vi "SSL UDP Receiver.vi"(11 "Cluster":T1) -> (0 "error out":errorcluster, 2 "RX":bool, 3 "data camera out":u8[](array[numeric]))   [LabVIEW 2020]
uses:
  Controls/vision_control.ctl
  <vilib>/Utility/tcp.llb/UDP Multicast Read-Only Open.vi
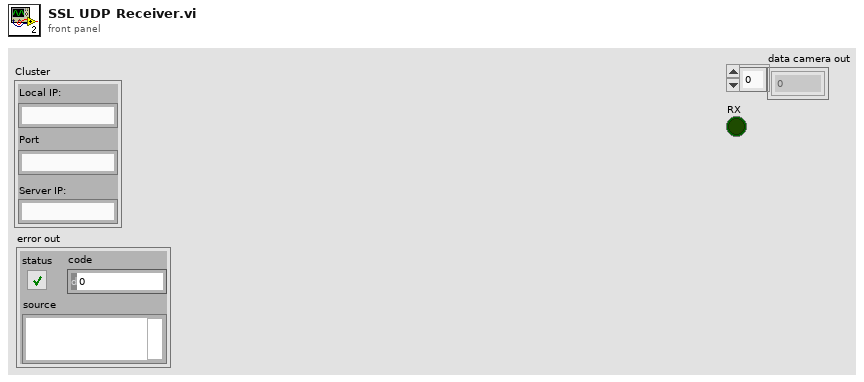
[diagram p1: front panel]
types:
  T1 = typedef "vision_control.ctl" = cluster{"Local IP:":string, "Server IP:":string, "Port":string}
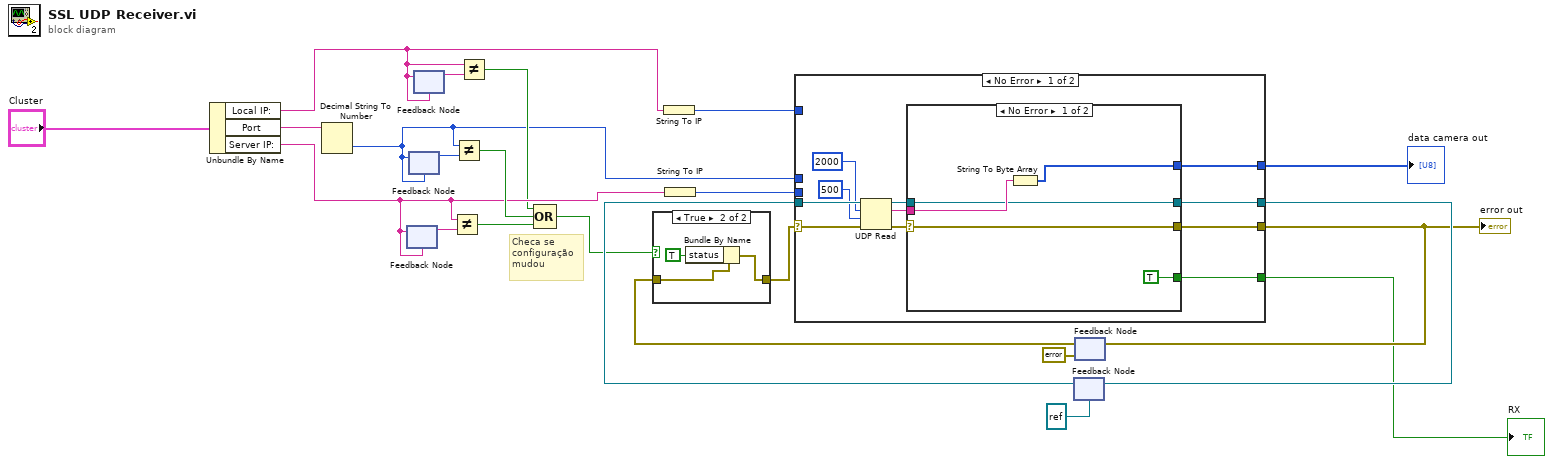
[diagram p0: block diagram]
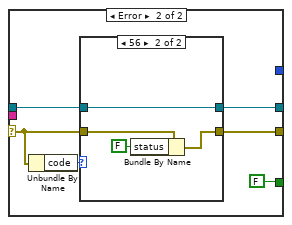
[diagram p3: hidden frame]
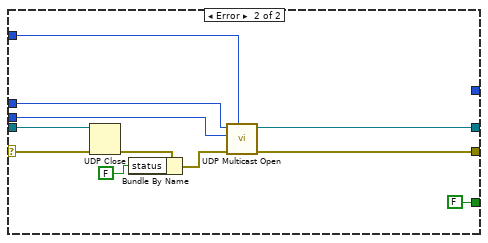
[diagram p5: hidden frame]
diagram:
  # "Checa se \nconfiguração\nmudou"
  n1 = Unbundle By Name("Cluster") -> ("Local IP:"=w8:string, "Port"=w2:string, "Server IP:"=w11:string)
  n2 = Decimal String To Number(string=w2) -> (number=w1:i32)  [unwired: 2 in, 1 out]
  n3 = feedback-in #1(w11) -> ()
  n4 = feedback #1(w11) -> (w16:string)
  n5 = feedback #2(w1) -> (w14:i32)
  n6 = feedback-in #2(w1) -> ()
  n7 = feedback #3(w8) -> (w10:string)
  n8 = feedback-in #3(w8) -> ()
  n9 = Not Equal?(x=w11, y=w16) -> (x != y?=w15:bool)
  n10 = Not Equal?(x=w1, y=w14) -> (x != y?=w13:bool)
  n11 = Not Equal?(x=w8, y=w10) -> (x != y?=w9:bool)
  n12 = Compound Arithmetic op=OR(w9, w13, w15) -> (w12:bool)
  n13 = String To IP(1:w8) -> (0:w7:u32)
  n14 = String To IP(1:w11) -> (0:w21:u32)
  n15 = feedback #4(refnum<k16> refnum ("connection ID")) -> (w22:refnum<k16>)
  n16 = feedback #5(errorcluster {"status"=TRUE, "code"=0, "source"=""} ("error out")) -> (w18:errorcluster)
  n17 = case shown="True" w12 {
    tunnel: w18 -> [w24 w26]
    tunnel: [w24 w25] -> w17
    frame False {
    }
    frame True {
      n18 = Bundle By Name(cluster=w26, "status"=TRUE) -> (w25:errorcluster)
    }
  }
  n19 = case shown="No Error" w17 {
    selector: w17 -> [w29 w57]
    tunnel: w22 -> [w38 w63]
    tunnel: [w37 w65] -> w6
    tunnel: [w36 w66] -> w23
    tunnel: w1 -> [_ w64]
    tunnel: w21 -> [_ w62]
    tunnel: [w30 FALSE] -> w3
    tunnel: w7 -> [_ w56]
    tunnel: [w28 _] -> w4
    frame No Error {
      n20 = UDP Read(connection ID=w38, max size (548)=2000, timeout ms (25000)=500, 8:w29) -> (data out=w33:string, error out=w31:errorcluster, 3:w32:refnum<k16>)  [unwired: 2 out]
      n21 = case shown="No Error" w31 {
        selector: w31 -> [w40 w44]
        tunnel: w33 -> [w43 _]
        tunnel: [w40 w46] -> w37
        tunnel: [w42 w47] -> w36
        tunnel: w32 -> [w42 w48]
        tunnel: [TRUE FALSE] -> w30
        tunnel: [w39 _] -> w28
        frame No Error {
          n22 = String To Byte Array(string=w43) -> (unsigned byte array=w39:u8[])
        }
        frame Error {
          n23 = Unbundle By Name(w44) -> ("code"=w49:i32)
          n24 = case shown="56" w49 {
            tunnel: w44 -> [w51 w55]
            tunnel: [w51 w53] -> w46
            tunnel: w48 -> [w50 w52]
            tunnel: [w50 w52] -> w47
            frame Default {
            }
            frame 56 {
              n25 = Bundle By Name(cluster=w55, "status"=FALSE) -> (w53:errorcluster)
            }
          }
        }
      }
    }
    frame Error {
      n26 = UDP Close(connection ID=w63, 8:w57) -> (error out=w60:errorcluster)  [unwired: 1 out]
      n27 = Bundle By Name(cluster=w60, "status"=FALSE) -> (w58:errorcluster)
      n28 = call-poly <vilib>:"UDP Multicast Open.vi"("net address"=w56, "error in (no error)"=w58, "multicast addr"=w62, "port"=w64) -> ("error out"=w65:errorcluster, "connection ID"=w66:refnum<k16>)  [unwired: 5 in, 1 out]
    }
  }
  "error out" <- w6
  "data camera out" <- w4
  "RX" <- w3
  n29 = feedback-in #4(w23) -> ()
  n30 = feedback-in #5(w6) -> ()
